vi "Example Callback.vi"() -> ()   [LabVIEW 2013]
uses:
  C:/tf/play/labview/Tinkerforge.dll
  Tinkerforge.dll
panel:
  out "logitude (°)":string
  out "latitude (°)":string
  in  "stop":bool
  in  "uid":string="21Kf"
  in  "port":i32=4223
  in  "host":string="localhost"
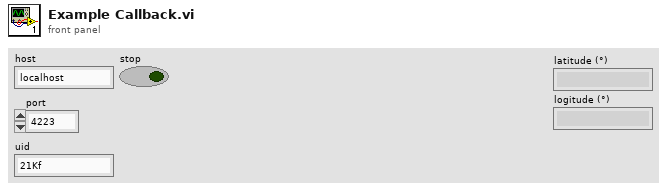
[diagram p1: front panel]
types:
  T1 = cluster{"latitude":i64, "ns":u16, "longitude":i64, "ew":u16}
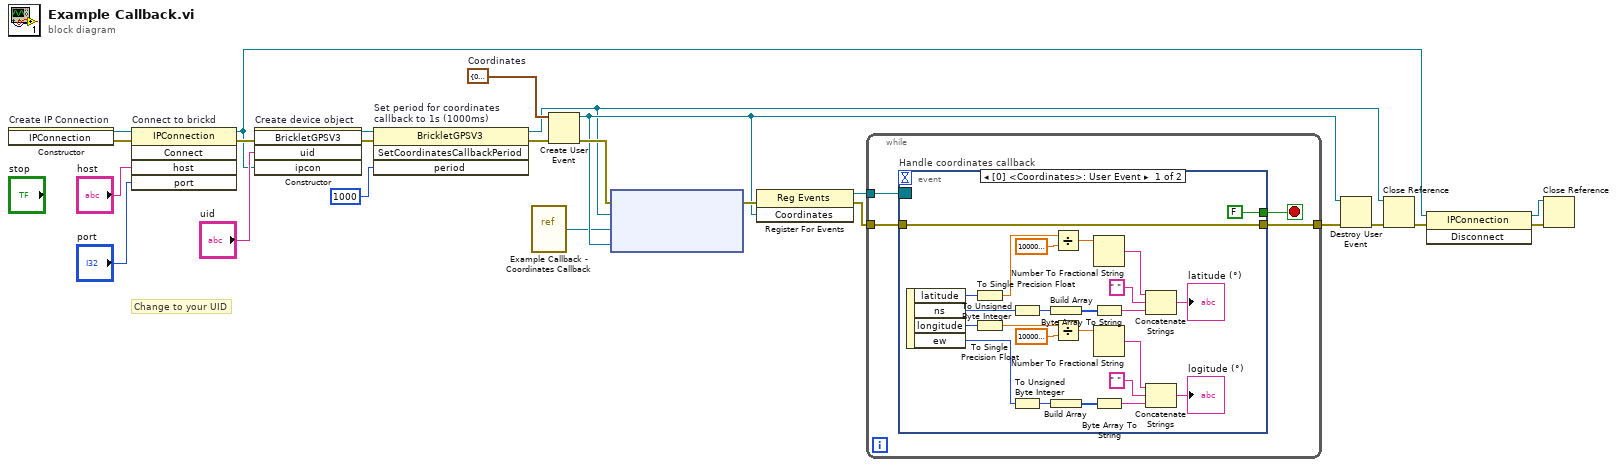
[diagram p0: block diagram]
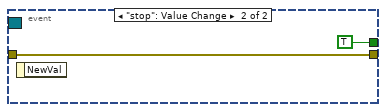
[diagram p2: hidden frame]
diagram:
  w8 = T1 {"latitude"=0, "ns"=0, "longitude"=0, "ew"=0}  # Coordinates
  # "Change to your UID"
  n1 = constructor on="Create IP Connection" class="IPConnection"() -> (reference out=w24:refnum<k24>, error out=w2:errorcluster)  [unwired: 3 in, 1 out]
  n2 = invoke on="Connect to brickd" class="IPConnection" method="Connect"(reference=w24, error in=w2, "host"="host", "port"="port") -> (reference out=w17:refnum<k24>, error out=w20:errorcluster)  [unwired: 1 in, 3 out]
  n3 = constructor on="Create device object" class="BrickletGPSV3"(error in=w20, "uid"="uid", "ipcon"=w17) -> (reference out=w5:refnum<k24>, error out=w7:errorcluster)  [unwired: 2 in, 3 out]
  n4 = invoke on="Set period for coordinates\ncallback to 1s (1000ms)" class="BrickletGPSV3" method="SetCoordinatesCallbackPeriod"(reference=w5, error in=w7, "period"=i64 1000) -> (reference out=w4:refnum<k24>, error out=w6:errorcluster)  [unwired: 1 in, 2 out]
  n5 = vi-ref "Example Callback - Coordinates Callback.vi"() -> ("vi reference"=w1:refnum<vi>)
  n6 = Create User Event(user event datatype=w8, error in=w6) -> (user event=w10:refnum<user-event>, error out=w15:errorcluster)
  n7 = node ("Register Event Callback")(w15, w4, w1, w10) -> (w14:errorcluster)  [unwired: 1 in, 1 out]
  n8 = register-events(error in=w14, w10) -> (reference out=w13:refnum<event-registration>, error out=w11:errorcluster)  [unwired: 1 in]
  n9 = while {
    tunnel: w13 -> [w28]
    tunnel: [w27] -> w12
    tunnel: w11 -> [w26]
    stop <- w25 stop-if-true
    n10 = event "Handle coordinates callback" shown="[0] <Coordinates>: User Event" {
      selector: w28 -> [_ _]
      dyn-events: _ -> [_ _]
      timeout: _ -> [_ _]
      tunnel: [w52 w53] -> w27
      tunnel: w26 -> [w52 w53]
      tunnel: [FALSE TRUE] -> w25
      event User Event {
        n11 = event-data() -> ("latitude"=w42:i64, "ns"=w41:u16, "longitude"=w31:i64, "ew"=w30:u16)  [unwired: 1 in]
        n12 = To Single Precision Float(number=w42) -> (single precision float=w50:sgl)
        n13 = To Single Precision Float(number=w31) -> (single precision float=w39:sgl)
        n14 = To Unsigned Byte Integer(number=w41) -> (unsigned 8bit integer=w47:u8)
        n15 = To Unsigned Byte Integer(number=w30) -> (unsigned 8bit integer=w36:u8)
        n16 = Build Array(w47) -> (w48:u8[])
        n17 = Build Array(w36) -> (w37:u8[])
        n18 = Divide(x=w50, y=sgl 1000000.0) -> (x/y=w43:sgl)
        n19 = Divide(x=w39, y=sgl 1000000.0) -> (x/y=w32:sgl)
        n20 = Number To Fractional String(number=w43) -> (F-format string=w44:string)  [unwired: 3 in]
        n21 = Byte Array To String(unsigned byte array=w48) -> (string=w45:string)
        n22 = Number To Fractional String(number=w32) -> (F-format string=w33:string)  [unwired: 3 in]
        n23 = Byte Array To String(unsigned byte array=w37) -> (string=w34:string)
        n24 = Concatenate Strings(w44, " ", w45) -> (→"latitude (°)":string)
        n25 = Concatenate Strings(w33, " ", w34) -> (→"logitude (°)":string)
      }
      event "stop": Value Change {
        n26 = event-data() -> ()  [unwired: 1 in, 1 out]
      }
    }
  }
  n27 = Destroy User Event(user event=w10, error in=w12) -> (error out=w9:errorcluster)
  n28 = Close Reference(reference=w4, error in (no error)=w9) -> (error out=w19:errorcluster)
  n29 = invoke class="IPConnection" method="Disconnect"(reference=w17, error in=w19) -> (reference out=w16:refnum<k24>, error out=w18:errorcluster)  [unwired: 1 in, 1 out]
  n30 = Close Reference(reference=w16, error in (no error)=w18) -> ()  [unwired: 1 out]
